vi "Determine Warnings 3.vi"() -> ()   [LabVIEW 2014]
panel:
  out "Warning?":bool
  out "Warning Text":string
  in  "Max Temp":dbl
  in  "Min Temp":dbl
  in  "Current Temp":dbl
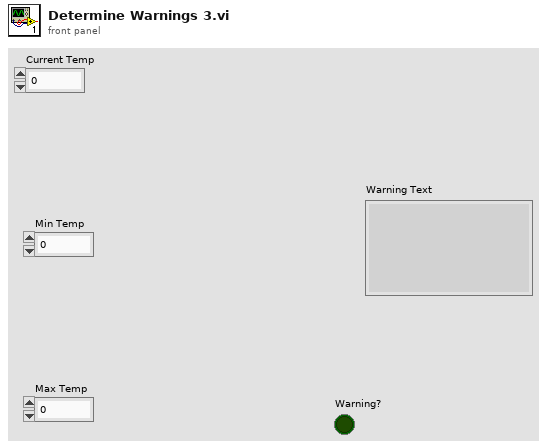
[diagram p1: front panel]
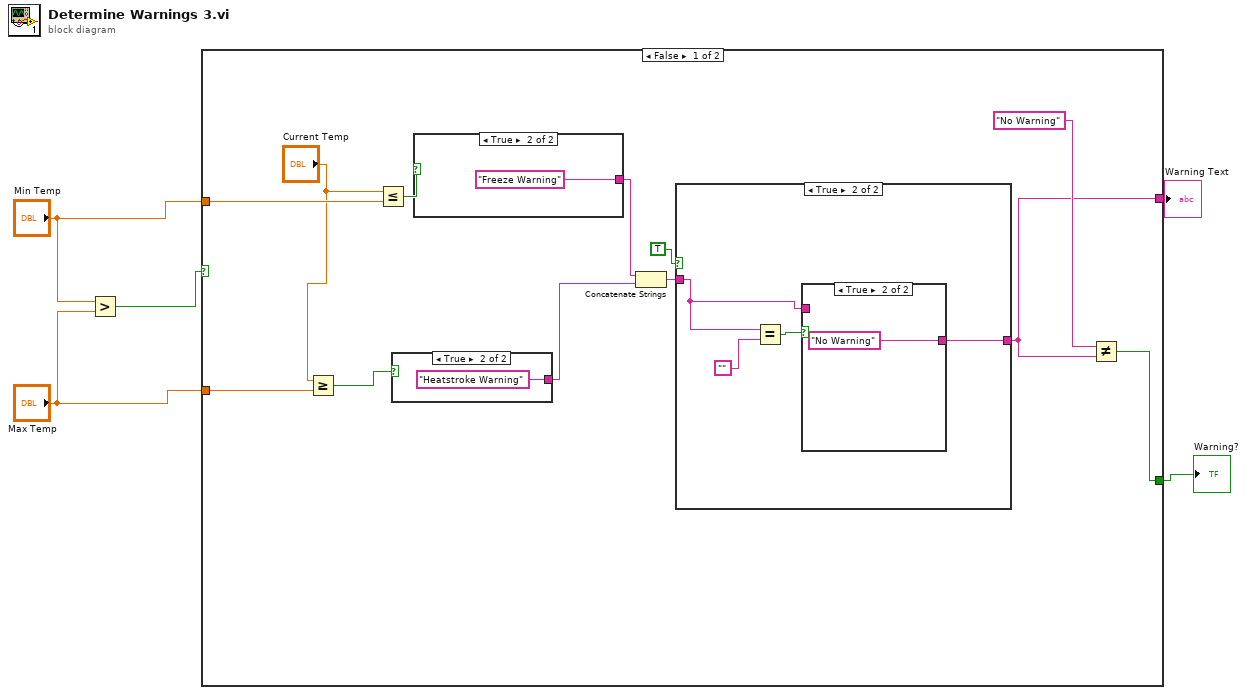
[diagram p0: block diagram]
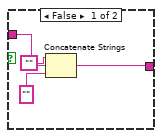
[diagram p3: hidden frame]
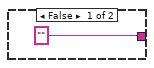
[diagram p4: hidden frame]
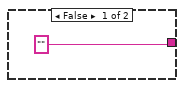
[diagram p5: hidden frame]
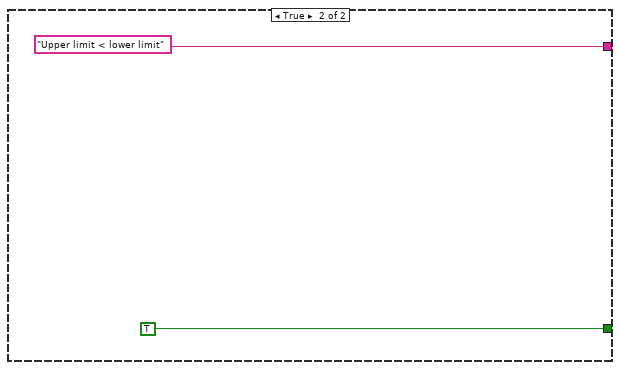
[diagram p6: hidden frame]
diagram:
  n1 = Greater?(x="Min Temp", y="Max Temp") -> (0:w2:bool)
  n2 = case shown="False" w2 {
    tunnel: "Min Temp" -> [w17 _]
    tunnel: "Max Temp" -> [w16 _]
    tunnel: [w7 "Upper limit < lower limit"] -> w5
    tunnel: [w6 TRUE ("Warning?")] -> w1
    frame False {
      n3 = Greater Or Equal?(x="Current Temp", y=w16) -> (x >= y?=w13:bool)
      n4 = Less Or Equal?(x="Current Temp", y=w17) -> (x <= y?=w14:bool)
      n5 = case shown="True" w13 {
        tunnel: ["" "Heatstroke Warning"] -> w10
        frame False {
        }
        frame True {
        }
      }
      n6 = case shown="True" w14 {
        tunnel: ["" "Freeze Warning"] -> w11
        frame False {
        }
        frame True {
        }
      }
      n7 = Concatenate Strings(w11, w10) -> (w12:string)
      n8 = case shown="True" TRUE {
        tunnel: w12 -> [w18 w20]
        tunnel: [w18 w19] -> w7
        frame False {
        }
        frame True {
          n9 = Equal?(x=w20, y="") -> (x = y?=w21:bool)
          n10 = case shown="True" w21 {
            tunnel: w20 -> [w25 _]
            tunnel: [w23 "No Warning"] -> w19
            frame False {
              n11 = Concatenate Strings("", w25, "") -> (w23:string)
            }
            frame True {
            }
          }
        }
      }
      n12 = Not Equal?(x="No Warning", y=w7) -> (x != y?=w6:bool)
    }
    frame True {
    }
  }
  "Warning Text" <- w5
  "Warning?" <- w1
